vi "GetModuleInfo.vi"(8 "error in (no error)":errorcluster, 10 "SN Number":string[](array[string]), 11 "Target (localhost)":refnum<k21>="localhost") -> (0 "error out":errorcluster, 2 "Modules":T1[](array[typedef]))   [LabVIEW 2017, in "TSNcDAQ_AI.lvlib"]
uses:
  <vilib>/addons/InsightCM/Devices/Shared/Cms/DAQmx/TSNcDAQ_AI.lvlib
  <vilib>/addons/cRIODetectHW/control/cRIO Product Info.ctl
  <vilib>/nisyscfg/Close (System).vi
  <vilib>/nisyscfg/nisyscfg.lvlib
  <resource>/objmgr/niflexrioatomicsae.rc
  <vilib>/addons/cRIODetectHW/cRIODetectHW.lvlib
  <resource>/objmgr/nicontrollersysapi.rc
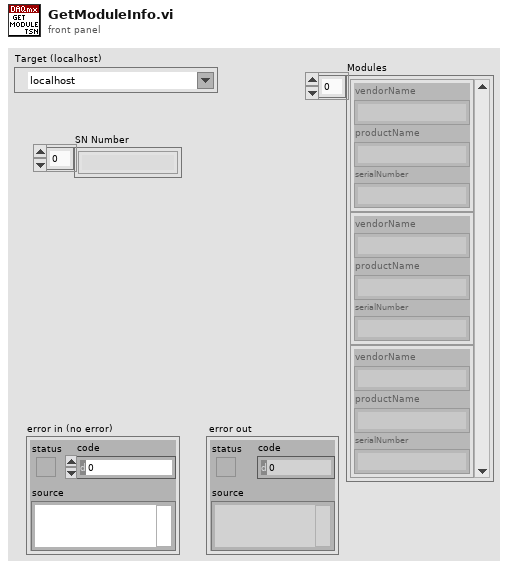
[diagram p1: front panel]
types:
  T1 = typedef "cRIODetectHW.lvlib/cRIO Product Info.ctl" = cluster{"vendorName":string, "productName":string, "serialNumber":string}
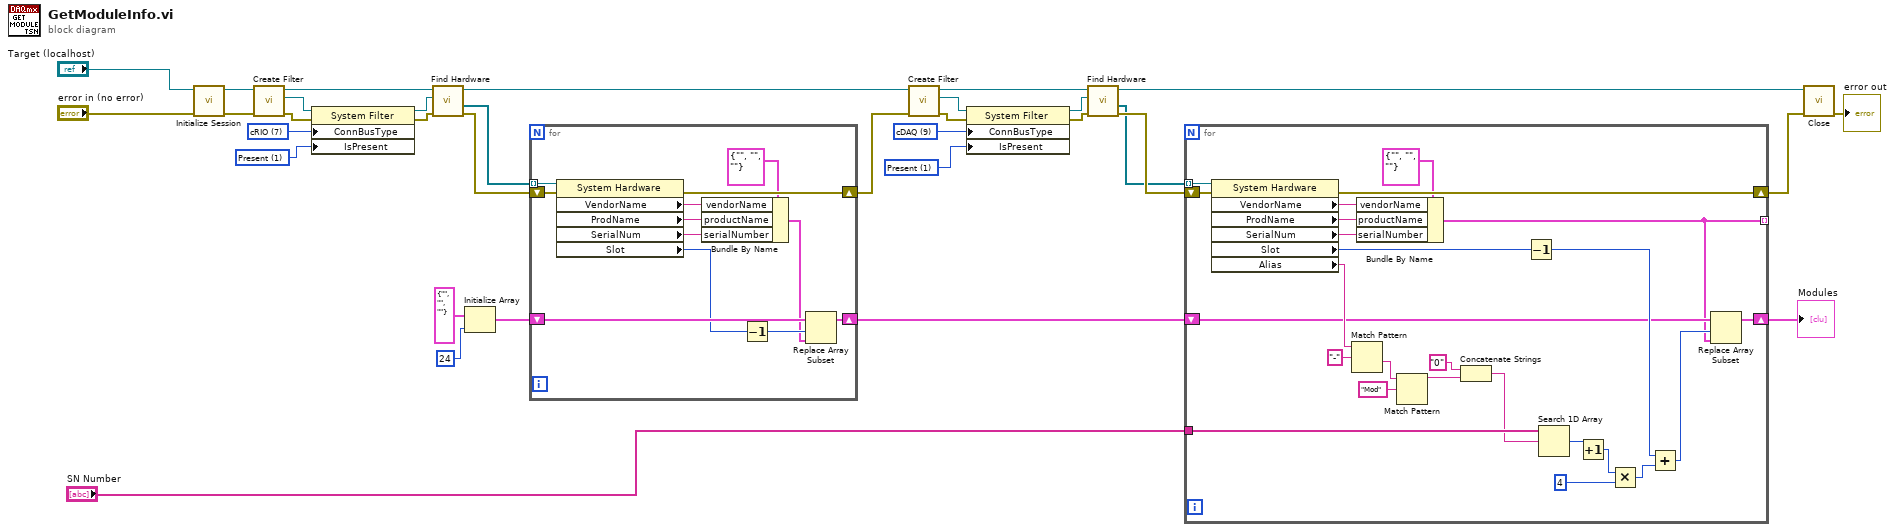
[diagram p0: block diagram]
diagram:
  w32 = 1 items=["Initializing"=-2, "Unknown"=-1, "Not Present"=0, "Present"=1] ("Devices & Chassis:Is Present")
  w31 = 1 items=["Initializing"=-2, "Unknown"=-1, "Not Present"=0, "Present"=1] ("Devices & Chassis:Is Present")
  w23 = u32 7 items=["BuiltIn/System", "PXI/PCI", "USB", "GPIB", "VXI", "Serial", "TCP/IP", "cRIO", "SCXI", "cDAQ", "SwitchBlock", "SCC", "FireWire", "Accessory", "CAN", "SwitchBlock Device"] ("Devices & Chassis:Connects To Bus Type")
  w6 = u32 9 items=["BuiltIn/System", "PXI/PCI", "USB", "GPIB", "VXI", "Serial", "TCP/IP", "cRIO", "SCXI", "cDAQ", "SwitchBlock", "SCC", "FireWire", "Accessory", "CAN", "SwitchBlock Device"] ("Devices & Chassis:Connects To Bus Type")
  n1 = call <vilib>:"Initialize Session.vi"("error in (no error)"="error in (no error)", "Target (localhost)"="Target (localhost)") -> ("error out"=w4:errorcluster, "Session out"=w5:refnum<k21>)  [unwired: 8 in]
  n2 = call <vilib>:"Create Filter.vi"("error in (no error)"=w4, "Session in"=w5) -> ("error out"=w19:errorcluster, "Filter out"=w20:refnum<k20>, "Session out"=w21:refnum<k21>)  [unwired: 7 in]
  n3 = property class="System Filter"(reference=w20, error in=w19, "ConnBusType"=w23, "IsPresent"=w32) -> (reference out=w22:refnum<k20>, error out=w18:errorcluster)
  n4 = call <vilib>:"Find Hardware.vi"("error in (no error)"=w18, "Filter in"=w22, "Session in"=w21) -> ("error out"=w16:errorcluster, "Resources out"=w17:refnum<k20>[], "Session out"=w24:refnum<k21>)  [unwired: 1 in, 5 out]
  n5 = Initialize Array(T1 {"vendorName"="", "productName"="", "serialNumber"=""} ("cRIO Module Info"), 24 ("dimension size")) -> (w28:T1[])
  n6 = for {
    tunnel: w17 -> [w45] mode=indexing
    shift-right: [w43] -> w25
    shift-left: w16 -> [w44]
    shift-right: [w34] -> w29
    shift-left: w28 -> [w38]
    n7 = property class="System Hardware"(reference=w45, error in=w44) -> (error out=w43:errorcluster, "VendorName"=w42:string, "ProdName"=w41:string, "SerialNum"=w40:string, "Slot"=w37:i32)  [unwired: 1 out]
    n8 = Bundle By Name(cluster=T1 {"vendorName"="", "productName"="", "serialNumber"=""} ("cRIO Module Info"), "vendorName"=w42, "productName"=w41, "serialNumber"=w40) -> (w35:T1)
    n9 = Decrement(x=w37) -> (x-1=w36:i32)
    n10 = Replace Array Subset(array=w38, new element=w35, index=w36) -> (w34:T1[])
  }
  n11 = call <vilib>:"Create Filter.vi"("error in (no error)"=w25, "Session in"=w24) -> ("error out"=w11:errorcluster, "Filter out"=w9:refnum<k20>, "Session out"=w8:refnum<k21>)  [unwired: 7 in]
  n12 = property class="System Filter"(reference=w9, error in=w11, "ConnBusType"=w6, "IsPresent"=w31) -> (reference out=w7:refnum<k20>, error out=w12:errorcluster)
  n13 = call <vilib>:"Find Hardware.vi"("error in (no error)"=w12, "Filter in"=w7, "Session in"=w8) -> ("error out"=w14:errorcluster, "Resources out"=w13:refnum<k20>[], "Session out"=w10:refnum<k21>)  [unwired: 1 in, 5 out]
  n14 = for {
    tunnel: w13 -> [w70] mode=indexing
    shift-right: [w68] -> w15
    shift-left: w14 -> [w69]
    tunnel: [w49] -> _ mode=indexing
    tunnel: "SN Number" -> [w59]
    shift-right: [w52] -> w30
    shift-left: w29 -> [w51]
    n15 = property class="System Hardware"(reference=w70, error in=w69) -> (error out=w68:errorcluster, "VendorName"=w67:string, "ProdName"=w66:string, "SerialNum"=w65:string, "Slot"=w55:i32, "Alias"=w63:string)  [unwired: 1 out]
    n16 = Match Pattern(string=w63, regular expression="-") -> (after substring=w61:string)  [unwired: 1 in, 3 out]
    n17 = Bundle By Name(cluster=T1 {"vendorName"="", "productName"="", "serialNumber"=""} ("cRIO Module Info"), "vendorName"=w67, "productName"=w66, "serialNumber"=w65) -> (w49:T1)
    n18 = Match Pattern(string=w61, regular expression="Mod") -> (before substring=w48:string)  [unwired: 1 in, 3 out]
    n19 = Concatenate Strings("0" ("string"), w48) -> (w46:string)
    n20 = Decrement(x=w55) -> (x-1=w53:i32)
    n21 = Search 1D Array(1D array=w59, element=w46) -> (index of element=w58:i32)  [unwired: 1 in]
    n22 = Increment(x=w58) -> (x+1=w56:i32)
    n23 = Multiply(x=w56, y=4) -> (x*y=w54:i32)
    n24 = Add(x=w53, y=w54) -> (x+y=w50:i32)
    n25 = Replace Array Subset(array=w51, new element=w49, index=w50) -> (w52:T1[])
  }
  "Modules" <- w30
  n26 = call-poly <vilib>:"Close.vi"("error in (no error)"=w15, "Session in"=w10) -> ("error out"=→"error out":errorcluster)  [unwired: 9 in]
